vi "Configure List.vi"(0 "VISA resource name":refnum<visa-resource-name>, 5 "Operation Mode (0: Current)":u16(ring) items=["Current", "Voltage", "Resistance", "Power"], 7 "LIST Array":dbl[][](array[numeric])=[[0.0, 0.0, 0.0, 0.0, 0.0], [0.0, 0.0, 0.0, 0.0, 0.0]] min=0.0 max=800000.0, 9 "Sampling (F)":bool, 11 "error in (no error)":errorcluster, 12 "Execution Mode (0: Loops)":u16(ring) items=["Loops", "Continuously"], 13 "Loops (1)":u32=1 min=1 max=4000000000 step=1) -> (4 "VISA resource name out":refnum<visa-resource-name>, 15 "error out":errorcluster)   [LabVIEW 2017, in "HH PLI Series.lvlib"]
doc: "Configures a free definable list of points.\n\n<b>Note</b>\nThe list points are limited to 300.\nUse a column-dimension of 5 for the List Array.\nRefer to instrument manual for details."
uses:
  HH PLI Series.lvlib
panel:
  # "I/V/Ohm/W"
  # "Ramp Time"
  # "Dwell Time"
  # "s"
  # "Ramp Time           \n[s]"
  # "Dwell Time           \n[s]"
  # "Setting value           \n[A],[V],\n[Ohm],[W]"
  # "Sampling Time"
  # "Ramp           \n[s]"
  # "Dwell           \n[s]"
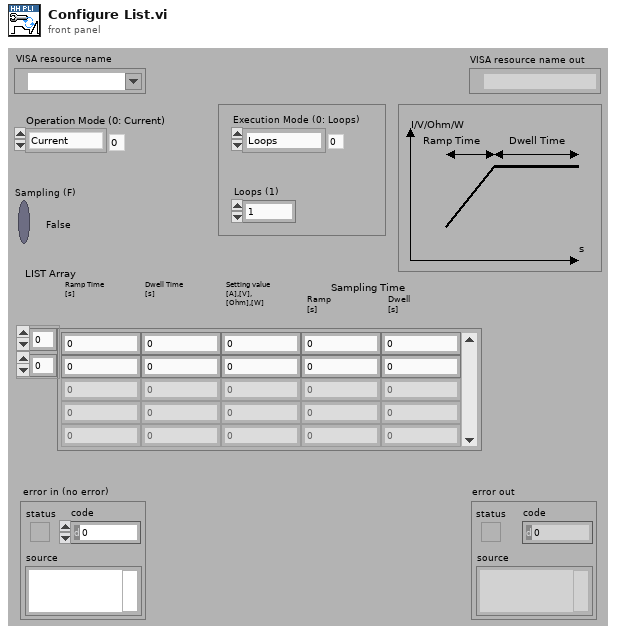
[diagram p1: front panel]
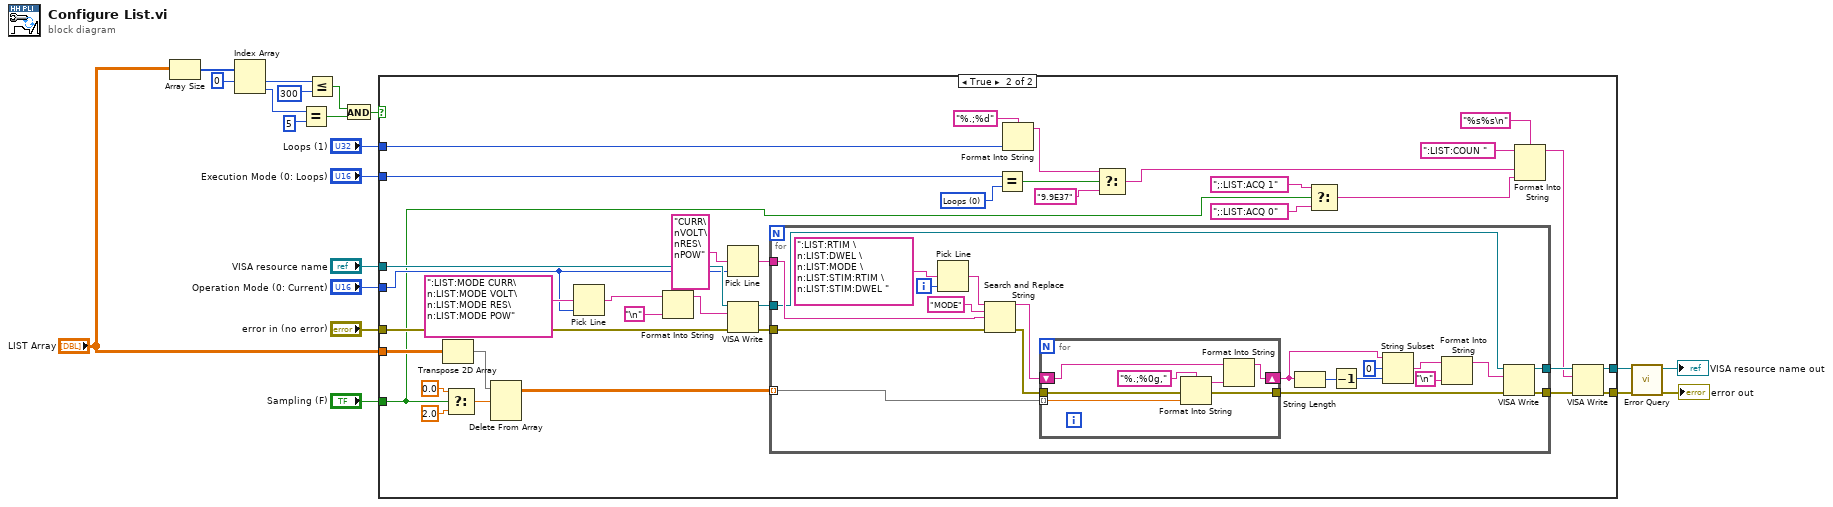
[diagram p0: block diagram]
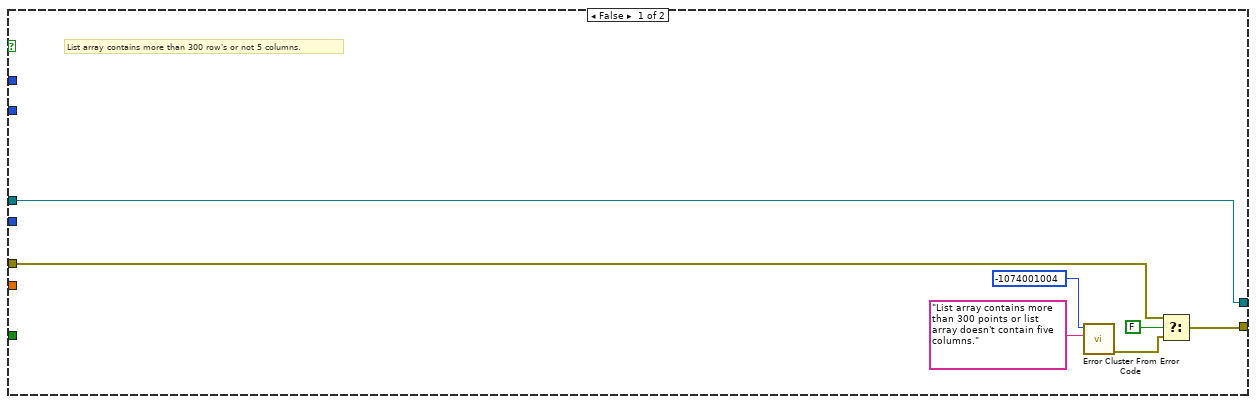
[diagram p2: hidden frame]
diagram:
  n1 = Array Size(array="LIST Array") -> (size(s)=w18:i32[])
  n2 = Index Array(array=w18, index #1=0 ("index")) -> (element #1=w16:i32, element #2=w6:i32)  [unwired: 1 in]
  n3 = Equal?(x=w6, y=5) -> (x = y?=w4:bool)
  n4 = Less Or Equal?(x=w16, y=300) -> (x <= y?=w3:bool)
  n5 = And(x=w3, y=w4) -> (x .and. y?=w5:bool)
  n6 = case shown="True" w5 {
    tunnel: "LIST Array" -> [_ w56]
    tunnel: "Sampling (F)" -> [_ w32]
    tunnel: "error in (no error)" -> [w22 w44]
    tunnel: [w21 w49] -> w13
    tunnel: "VISA resource name" -> [w27 w46]
    tunnel: [w27 w48] -> w10
    tunnel: "Execution Mode (0: Loops)" -> [_ w36]
    tunnel: "Loops (1)" -> [_ w53]
    tunnel: "Operation Mode (0: Current)" -> [_ w42]
    frame False {
      # "List array contains more than 300 row's or not 5 columns."
      n7 = call <vilib>:"Error Cluster From Error Code.vi"("error message (\"\")"="List array contains more than 300 points or list array doesn't contain five columns." ("Source (VI Name)"), "error code (0)"=-1074001004 ("Code")) -> ("error out"=w23:errorcluster)  [unwired: 7 in]
      n8 = Select(t=w22, s=FALSE ("show call chain? (False)"), f=w23) -> (s? t:f=w21:errorcluster)
    }
    frame True {
      w38 = u16 0 items=["Loops", "Continuously"] ("Execution Mode (0: Loops)")
      n9 = Transpose 2D Array(2D array=w56) -> (transposed array=w63:dbl[][])
      n10 = Select(t=0.0, s=w32, f=2.0) -> (s? t:f=w61:dbl)
      n11 = Delete From Array(array=w63, length=w61) -> (array with subset deleted=w62:dbl[][])  [unwired: 2 in, 1 out]
      n12 = Pick Line(multi-line string=":LIST:MODE CURR\n:LIST:MODE VOLT\n:LIST:MODE RES\n:LIST:MODE POW", line index=w42) -> (output string=w39:string)  [unwired: 1 in]
      n13 = Format Into String(initial string=w39, "\n") -> (resulting string=w41:string)  [unwired: 2 in, 1 out]
      n14 = Pick Line(multi-line string="CURR\nVOLT\nRES\nPOW", line index=w42) -> (output string=w57:string)  [unwired: 1 in]
      n15 = VISA Write(VISA resource name=w46, write buffer=w41, error in (no error)=w44) -> (VISA resource name out=w45:refnum<visa-resource-name>, error out=w43:errorcluster)  [unwired: 1 out]
      n16 = for {
        tunnel: w62 -> [w64] mode=indexing
        tunnel: w57 -> [w79]
        tunnel: w43 -> [w73]
        tunnel: [w69] -> w50
        tunnel: w45 -> [w70]
        tunnel: [w68] -> w51
        i -> [w83]
        n17 = Pick Line(multi-line string=":LIST:RTIM \n:LIST:DWEL \n:LIST:MODE \n:LIST:STIM:RTIM \n:LIST:STIM:DWEL ", line index=w83) -> (output string=w81:string)  [unwired: 1 in]
        n18 = Search and Replace String(input string=w81, search string="MODE", replace string=w79, error in=w73) -> (result string=w78:string, error out=w72:errorcluster)  [unwired: 4 in, 2 out]
        n19 = for {
          tunnel: w64 -> [w84] mode=indexing
          shift-right: [w85] -> w77
          shift-left: w78 -> [w87]
          tunnel: w72 -> [w89]
          tunnel: [w88] -> w71
          n20 = Format Into String(format string="%.;%0g,", error in=w89, w84) -> (resulting string=w86:string, error out=w88:errorcluster)  [unwired: 1 in]
          n21 = Format Into String(initial string=w87, w86) -> (resulting string=w85:string)  [unwired: 2 in, 1 out]
        }
        n22 = String Length(string=w77) -> (length=w76:i32)
        n23 = Decrement(x=w76) -> (x-1=w75:i32)
        n24 = String Subset(string=w77, offset (0)=0, length (rest)=w75) -> (substring=w66:string)
        n25 = Format Into String(initial string=w66, "\n") -> (resulting string=w67:string)  [unwired: 2 in, 1 out]
        n26 = VISA Write(VISA resource name=w70, write buffer=w67, error in (no error)=w71) -> (VISA resource name out=w68:refnum<visa-resource-name>, error out=w69:errorcluster)  [unwired: 1 out]
      }
      n27 = Equal?(x=w36, y=w38) -> (x = y?=w37:bool)
      n28 = Format Into String(format string="%.;%d", w53) -> (resulting string=w54:string)  [unwired: 2 in, 1 out]
      n29 = Select(t=w54, s=w37, f="9.9E37") -> (s? t:f=w33:string)
      n30 = Select(t=";:LIST:ACQ 1" ("f"), s=w32, f=";:LIST:ACQ 0") -> (s? t:f=w29:string)
      n31 = Format Into String(format string="%s%s\n", initial string=":LIST:COUN " ("f"), w33, w29) -> (resulting string=w28:string)  [unwired: 1 in, 1 out]
      n32 = VISA Write(VISA resource name=w51, write buffer=w28, error in (no error)=w50) -> (VISA resource name out=w48:refnum<visa-resource-name>, error out=w49:errorcluster)  [unwired: 1 out]
    }
  }
  n33 = call "Error Query.vi"("error in (no error)"=w13, "VISA resource name"=w10) -> ("error out"=→"error out":errorcluster, "VISA resource name out"=→"VISA resource name out":refnum<visa-resource-name>)  [unwired: 6 in, 2 out]
